vi "Read measurement.vi"(8 "error in (no error)":errorcluster, 11 "AH2500A in":refnum<class "AH2500A.lvclass">) -> (0 "error out":errorcluster, 2 "measurement":T1, 3 "AH2500A out":refnum<class "AH2500A.lvclass">)   [LabVIEW 2019, in "AH2500A.lvclass"]
uses:
  AH2500A.lvclass
  Typedefs/AH2500A Measurement--Cluster.ctl
  AH2500A.lvclass/AH2500A.ctl
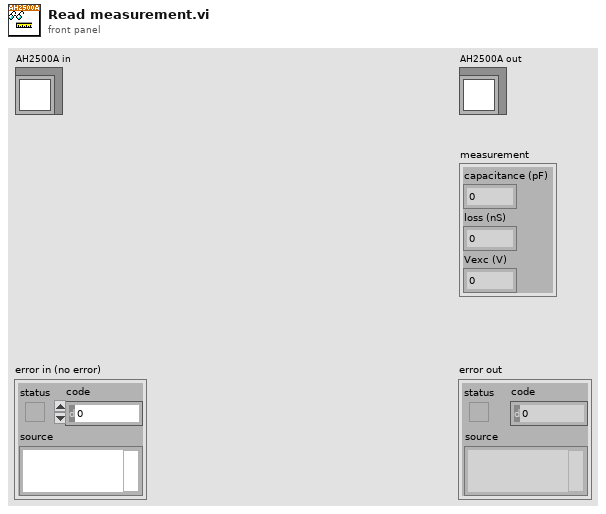
[diagram p1: front panel]
types:
  T1 = typedef "AH2500A.lvclass/AH2500A Measurement--Cluster.ctl" = cluster{"capacitance (pF)":dbl, "loss (nS)":dbl, "Vexc (V)":dbl}
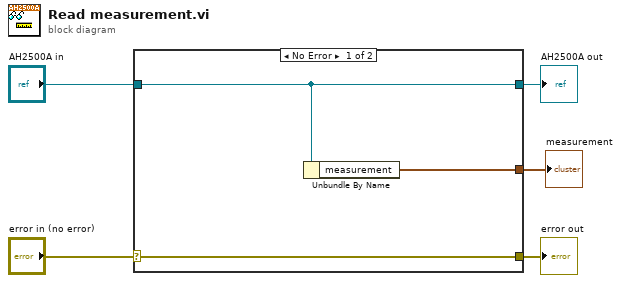
[diagram p0: block diagram]
diagram:
  n1 = case shown="No Error" "error in (no error)" {
    selector: "error in (no error)" -> [w8 w9]
    tunnel: [w8 w9] -> w4
    tunnel: [w6 w10] -> w2
    tunnel: "AH2500A in" -> [w6 w10]
    tunnel: [w7 _] -> w1
    frame No Error {
      n2 = Unbundle By Name(w6) -> ("measurement"=w7:T1)
    }
    frame Error {
    }
  }
  "error out" <- w4
  "AH2500A out" <- w2
  "measurement" <- w1
